vi "CAPTH Simulplot.vi"() -> ()   [LabVIEW 2020]
panel:
  out "AUDIOGRAM":cluster{dbl[], dbl[]}[](graph)=[{[44.07, 36.65, 30.49, 25.36, 21.09, 17.54, 14.59, 12.14, 10.1, 8.4, 6.98, 5.81, 4.83, 4.02, 3.34, 2.78, 2.31, 1.92, 0.0, 0.0], [63.95, 58.94, 57.98, 48.67, 43.89, 44.35, 35.31, 43.98, 47.28, 51.8, 60.32, 61.2, 60.22, 50.18, 45.97, 47.29, 47.2, 45.5, 0.0, 0.0]}, {[44.07, 36.65, 30.49, 25.36, 21.09, 17.54, 14.59, 12.14, 10.1, 8.4, 6.98, 5.81, 4.83, 4.02, 3.34, 2.78, 0.0, 0.0], [55.95, 56.94, 56.98, 43.67, 45.89, 42.35, 37.31, 42.98, 49.28, 49.8, 53.32, 51.2, 52.22, 48.18, 55.97, 50.29, 0.0, 0.0]}, {[44.07, 36.65, 30.49, 25.36, 21.09, 17.54, 14.59, 12.14, 10.1, 8.4, 6.98, 5.81, 4.83, 4.02, 3.34, 2.78, 0.0, 0.0], [52.95, 50.94, 47.98, 51.67, 47.89, 46.35, 37.31, 47.98, 51.28, 54.8, 51.32, 53.2, 49.22, 48.18, 41.97, 44.29, 0.0, 0.0]}, {[], []}]
  in  "?":u16(ring) items=["CAP FILE", "DP FILE"]
  out "?":string="2-9   \r2-1   \r2-0   \r"
  out "CAT":i32=2
  in  "Run# list: x;x;x":string="0;1;9;"
  in  "START":bool
  in  "RETURN":bool
  # "TYPE RUN#s HERE - xx;yy;zz"
  # "(max of 10)"
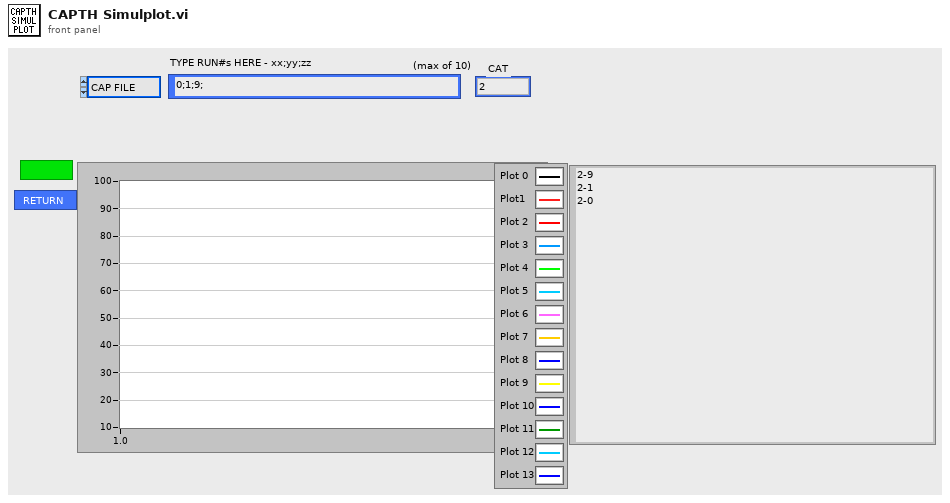
[diagram p1: front panel]
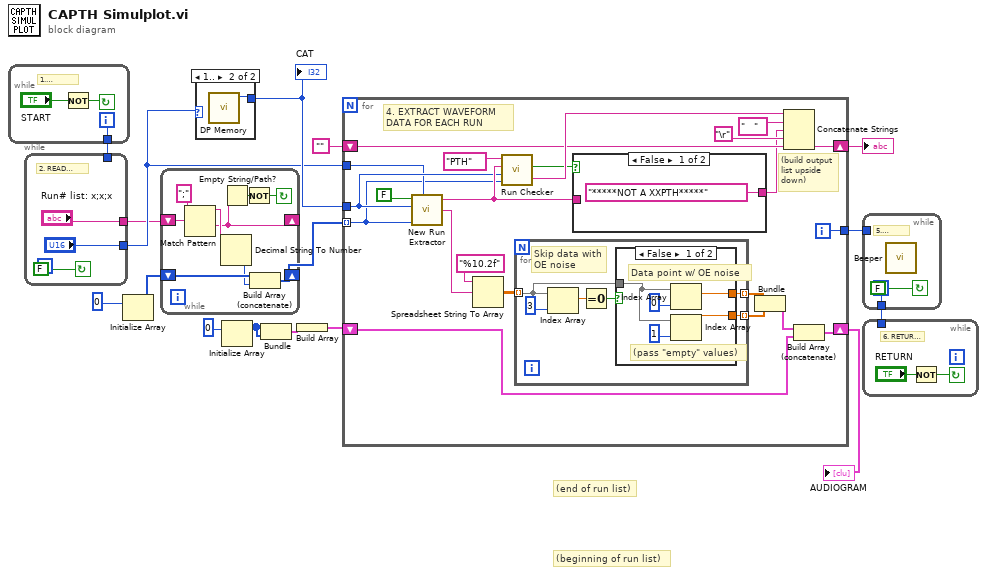
[diagram p0: block diagram]
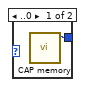
[diagram p2: hidden frame]
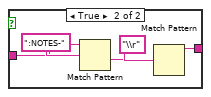
[diagram p3: hidden frame]
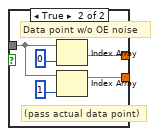
[diagram p4: hidden frame]
diagram:
  # "(beginning of run list)"
  # "(end of run list)"
  n1 = while {
    tunnel: [w17] -> w12
    i -> [w17]
    stop <- w18 continue-if-true
    # "1. STARTER"
    n2 = Not(x="START") -> (.not. x?=w18:bool)
  }
  n3 = while {
    tunnel: ["?"] -> w5
    tunnel: ["Run# list: x;x;x"] -> w4
    tunnel: w12 -> [_]
    stop <- FALSE continue-if-true
    # "2. READ INPUT"
  }
  n4 = Initialize Array(0) -> (w3:i32[])  [unwired: 1 in]
  n5 = while {
    shift-left: w3 -> [w31]
    shift-right: [w30] -> w1
    shift-left: w4 -> [w29]
    shift-right: [w25] -> _
    stop <- w23 continue-if-true
    n6 = Match Pattern(string=w29, regular expression=";") -> (before substring=w27:string, after substring=w25:string)  [unwired: 1 in, 2 out]
    n7 = Decimal String To Number(string=w27) -> (number=w26:i32)  [unwired: 2 in, 1 out]
    n8 = Empty String/Path?(string/path=w25) -> (empty?=w24:bool)
    n9 = Not(x=w24) -> (.not. x?=w23:bool)
    n10 = Build Array (concatenate)(w31, w26) -> (w30:i32[])
  }
  n11 = case shown="1.." w5 {
    tunnel: [w32 w33] -> w11
    frame ..0 {
      n12 = call "CAP memory.vi"() -> ("CN"=w32:u32)  [unwired: 6 in, 3 out]
    }
    frame 1.. {
      n13 = call "DP Memory.vi"() -> ("CURRENT Animal ID#"=w33:u32)  [unwired: 6 in, 2 out]
    }
  }
  "CAT" <- w11
  n14 = Initialize Array(0) -> (w7:i32[])  [unwired: 1 in]
  n15 = Bundle(w7, w7) -> (w9:cluster{i32[], i32[]})  [unwired: 1 in]
  n16 = Build Array(w9) -> (w8:cluster{i32[], i32[]}[])
  n17 = for {
    shift-right: [w53] -> w13
    shift-left: "" -> [w46]
    shift-right: [w37] -> w6
    shift-left: w8 -> [w36]
    tunnel: w11 -> [w43]
    tunnel: [w55] -> w16
    tunnel: w5 -> [w40]
    tunnel: w1 -> [w34] mode=indexing
    i -> [w55]
    # "4. EXTRACT WAVEFORM   DATA FOR EACH RUN"
    # "(build output list upside down)"
    n18 = call "New Run Extractor"("CAP (F) - SINGLE UNIT (T)"=FALSE, "Cat #"=w43, "Run #"=w34, "File Type CAP=0;DP=1)"=w40) -> ("HEADER STRING"=w44:string, "DATA STRING"=w42:string)  [unwired: 1 in, 1 out]
    n19 = Spreadsheet String To Array(format string="%10.2f", spreadsheet string=w42) -> (array=w49:dbl[][])  [unwired: 2 in]
    n20 = call "Run Checker"("RUN #"=w34, "UNIT #"=w43, "HEADER INPUT"=w44, "STRING TO MATCH"="PTH") -> ("STRING \"UN-RN\""=w51:string, "OK"=w41:bool)
    n21 = for {
      tunnel: [w62] -> w38 mode=indexing
      tunnel: [w63] -> w39 mode=indexing
      tunnel: w49 -> [w64] mode=indexing
      # "Skip data with OE noise"
      n22 = Index Array(array=w64, index=3) -> (element=w66:dbl)
      n23 = Equal To 0?(x=w66) -> (x = 0?=w65:bool)
      n24 = case shown="False" w65 {
        tunnel: [w69 w73] -> w62
        tunnel: [w70 w74] -> w63
        tunnel: w64 -> [w68 w75]
        frame False {
          # "(pass \"empty\" values)"
          # "Data point w/ OE noise"
          n25 = Index Array(array=w68, index=0) -> (element=w70:dbl)
          n26 = Index Array(array=w68, index=1) -> (element=w69:dbl)
        }
        frame True {
          # "(pass actual data point)"
          # "Data point w/o OE noise"
          n27 = Index Array(array=w75, index=0) -> (element=w74:dbl)
          n28 = Index Array(array=w75, index=1) -> (element=w73:dbl)
        }
      }
    }
    n29 = case shown="False" w41 {
      tunnel: w44 -> [_ w58]
      tunnel: ["*****NOT A XXPTH*****" w57] -> w45
      frame False {
      }
      frame True {
        n30 = Match Pattern(string=w58, regular expression=":NOTES-") -> (after substring=w60:string)  [unwired: 1 in, 3 out]
        n31 = Match Pattern(string=w60, regular expression="\\r") -> (before substring=w57:string)  [unwired: 1 in, 3 out]
      }
    }
    n32 = Bundle(w39, w38) -> (w35:cluster{dbl[], dbl[]})  [unwired: 1 in]
    n33 = Concatenate Strings(w51, "   ", w45, "\r", w46) -> (w53:string)
    n34 = Build Array (concatenate)(w35, w36) -> (w37:cluster{dbl[], dbl[]}[])
  }
  "?" <- w13
  "AUDIOGRAM" <- w6
  n35 = while {
    tunnel: w16 -> [_]
    tunnel: [w79] -> w15
    i -> [w79]
    stop <- FALSE continue-if-true
    # "5. SIGNAL"
    n36 = call "Beeper"() -> ()  [unwired: 1 in]
  }
  n37 = while {
    tunnel: w15 -> [_]
    stop <- w80 continue-if-true
    # "6. RETURN ?"
    n38 = Not(x="RETURN") -> (.not. x?=w80:bool)
  }
